vi "Thermistor_Extract.vi"(1 "Path":path, 2 "filenames":string[](array[string])) -> (0 "ThermTemps":dbl[](array[numeric]))   [LabVIEW 2022 SP3]
uses:
  <vilib>/Utility/file.llb/Read Delimited Spreadsheet (string).vi
panel:
  out "subarray":string[](array[string])
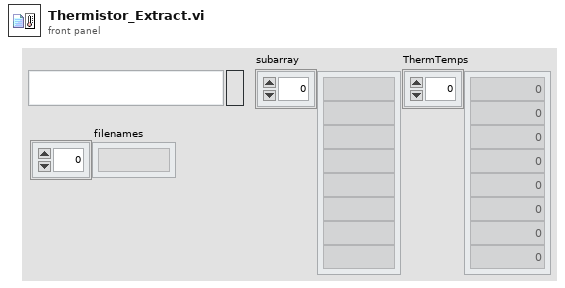
[diagram p1: front panel]
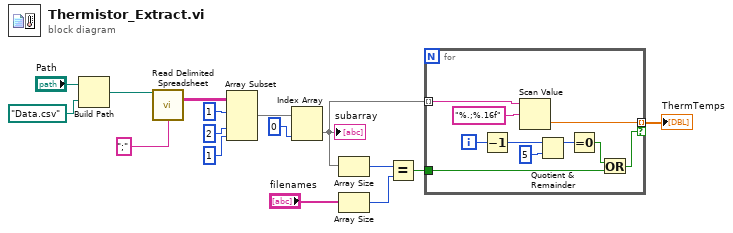
[diagram p0: block diagram]
diagram:
  n1 = Build Path(base path="Path", name or relative path=path "Data.csv") -> (appended path=w14:path)
  n2 = call-poly <vilib>:"Read Delimited Spreadsheet.vi"("file path (dialog if empty)"=w14, "delimiter (\\t)"=";" ("delimiter (\\t)")) -> ("all rows"=w12:string[][])  [unwired: 8 in, 5 out]
  n3 = Array Subset(array=w12, index (row)=1 ("index"), index (col)=2 ("index"), length (col)=1 ("length")) -> (w5:string[][])  [unwired: 1 in]
  n4 = Index Array(array=w5, index (col)=0 ("disabled index (col)")) -> (element=w2:string[])  [unwired: 1 in]
  "subarray" <- w2
  n5 = Array Size(array=w2) -> (size(s)=w4:i32)
  n6 = Array Size(array="filenames") -> (size(s)=w3:i32)
  n7 = Equal?(x=w4, y=w3) -> (x = y?=w1:bool)
  n8 = for {
    tunnel: w2 -> [w18] mode=indexing
    tunnel: [w17] -> w7 mode=indexing if=w21
    tunnel: w1 -> [w20]
    i -> [w26]
    n9 = Decrement(x=w26) -> (x-1=w22:i32)
    n10 = Scan Value(string=w18, format string="%.;%.16f") -> (value=w17:dbl)  [unwired: 1 in, 1 out]
    n11 = Quotient & Remainder(x=w22, y=5) -> (x-y*floor(x/y)=w24:i32)  [unwired: 1 out]
    n12 = Equal To 0?(x=w24) -> (x = 0?=w23:bool)
    n13 = Or(x=w23, y=w20) -> (x .or. y?=w21:bool)
  }
  "ThermTemps" <- w7
